vi "Wait and Monitor_UPS.vi"(8 "error in":errorcluster, 10 "Sequence Context":T3, 11 "WaitMoniter Input":T2={"Wait Time(S)"=10.0, "Chamber Temp(Deg C)"=10.0, "Chamber Temp Tolerance(%)"=10.0, "RMS Current(A)"=10.0, "RMS Current Tolerance(%)"=10.0, "Temperature Control"=FALSE, "RMS Control"=FALSE, "RMS Current Min(A)"=10.0, "RMS Current Max(A)"=10.0, "Chamber Temp Min(Deg C)"=10.0, "Chamber Temp Max(Deg C)"=10.0, "HVPPS Current Max(A)"=10.0, "HVPPS Control"=FALSE, "HVPPS Current(A)"=10.0} {"HVPPS Current(A)" format="%#_13g"; "HVPPS Current Max(A)" format="%#_13g"; "Chamber Temp Max(Deg C)" format="%#_13g"; "Chamber Temp Min(Deg C)" format="%#_13g"; "RMS Current Max(A)" format="%#_13g"; "RMS Current Min(A)" format="%#_13g"; "RMS Current Tolerance(%)" format="%#_13g"; "RMS Current(A)" format="%#_13g"; "Chamber Temp Tolerance(%)" format="%#_13g"; "Chamber Temp(Deg C)" format="%#_13g"; "Wait Time(S)" format="%#_13g"}) -> (0 "error out":errorcluster, 2 "Report Text":string, 3 "PowerMoniter out":refnum<class "Wait Monitor.lvclass">)   [LabVIEW 2023, in "HardwareAbstractionLayer_LVOOP.lvlib" / "Wait Monitor.lvclass"]
uses:
  Wait Monitor.lvclass
  <vilib>/addons/TestStand/_TSLegacy.llb/LabVIEW Test - Sequence Context.ctl
  Teststand Steptypes/WaitMoniter/Control/Moniter Step Control.ctl
  SubVI/Control/Data Cluster.ctl
  Teststand Steptypes/PowerMonitor/Control/PowerData.ctl
  SubVI/Control/TimerStates.ctl
  Teststand Steptypes/DAQ/Relay Output/Control/Relay Output.ctl
  <vilib>/addons/TestStand/_TSUtility.llb/TestStand - Get Property Value (Number {Unsigned 16-bit Integer}).vi
  Teststand Steptypes/GlobalVariable/GlobalVariableData.vi
  <vilib>/addons/TestStand/_TSUtility.llb/TestStand - Get Property Value (Number).vi
  <vilib>/addons/TestStand/_TSUtility.llb/TestStand - Set Property Value (Number).vi
  Teststand/Teststand.lvclass
  Teststand Steptypes/LTT_TeststandSteptypes.lvlib
  Database/Database.lvclass
  <userlib>/_OpenG.lib/error/error.llb/openg_error.lvlib
panel:
  out "RMS Refresh?":bool
  out "Elapsed Time":string
  out "HVPPS Current(A)":dbl[](array[numeric]) format="%#.3g"
  out "RTD Temp (Deg C)":dbl
  out "Raw Power":bool
  in  "Buzzer":bool
  out "RMS Current(A)":dbl[](array[numeric]) format="%#.3g"
  out "Target Temp (Deg C)":dbl
  out "Wait Time":string
  out "Current Time":string
  out "Remaining Time":string
  out "Enable Monitor":cluster{"RMS Current":bool, "Chamber":bool}
  out "Running Cycle":u16
  out "Test Mode":u16
  out "PPS Status":T1
  out "RunStates":string
  out "Status Update":string
  out "Elapsed time(S)":dbl format="%.1f"
  out "Chamber Temp(Deg C)":dbl
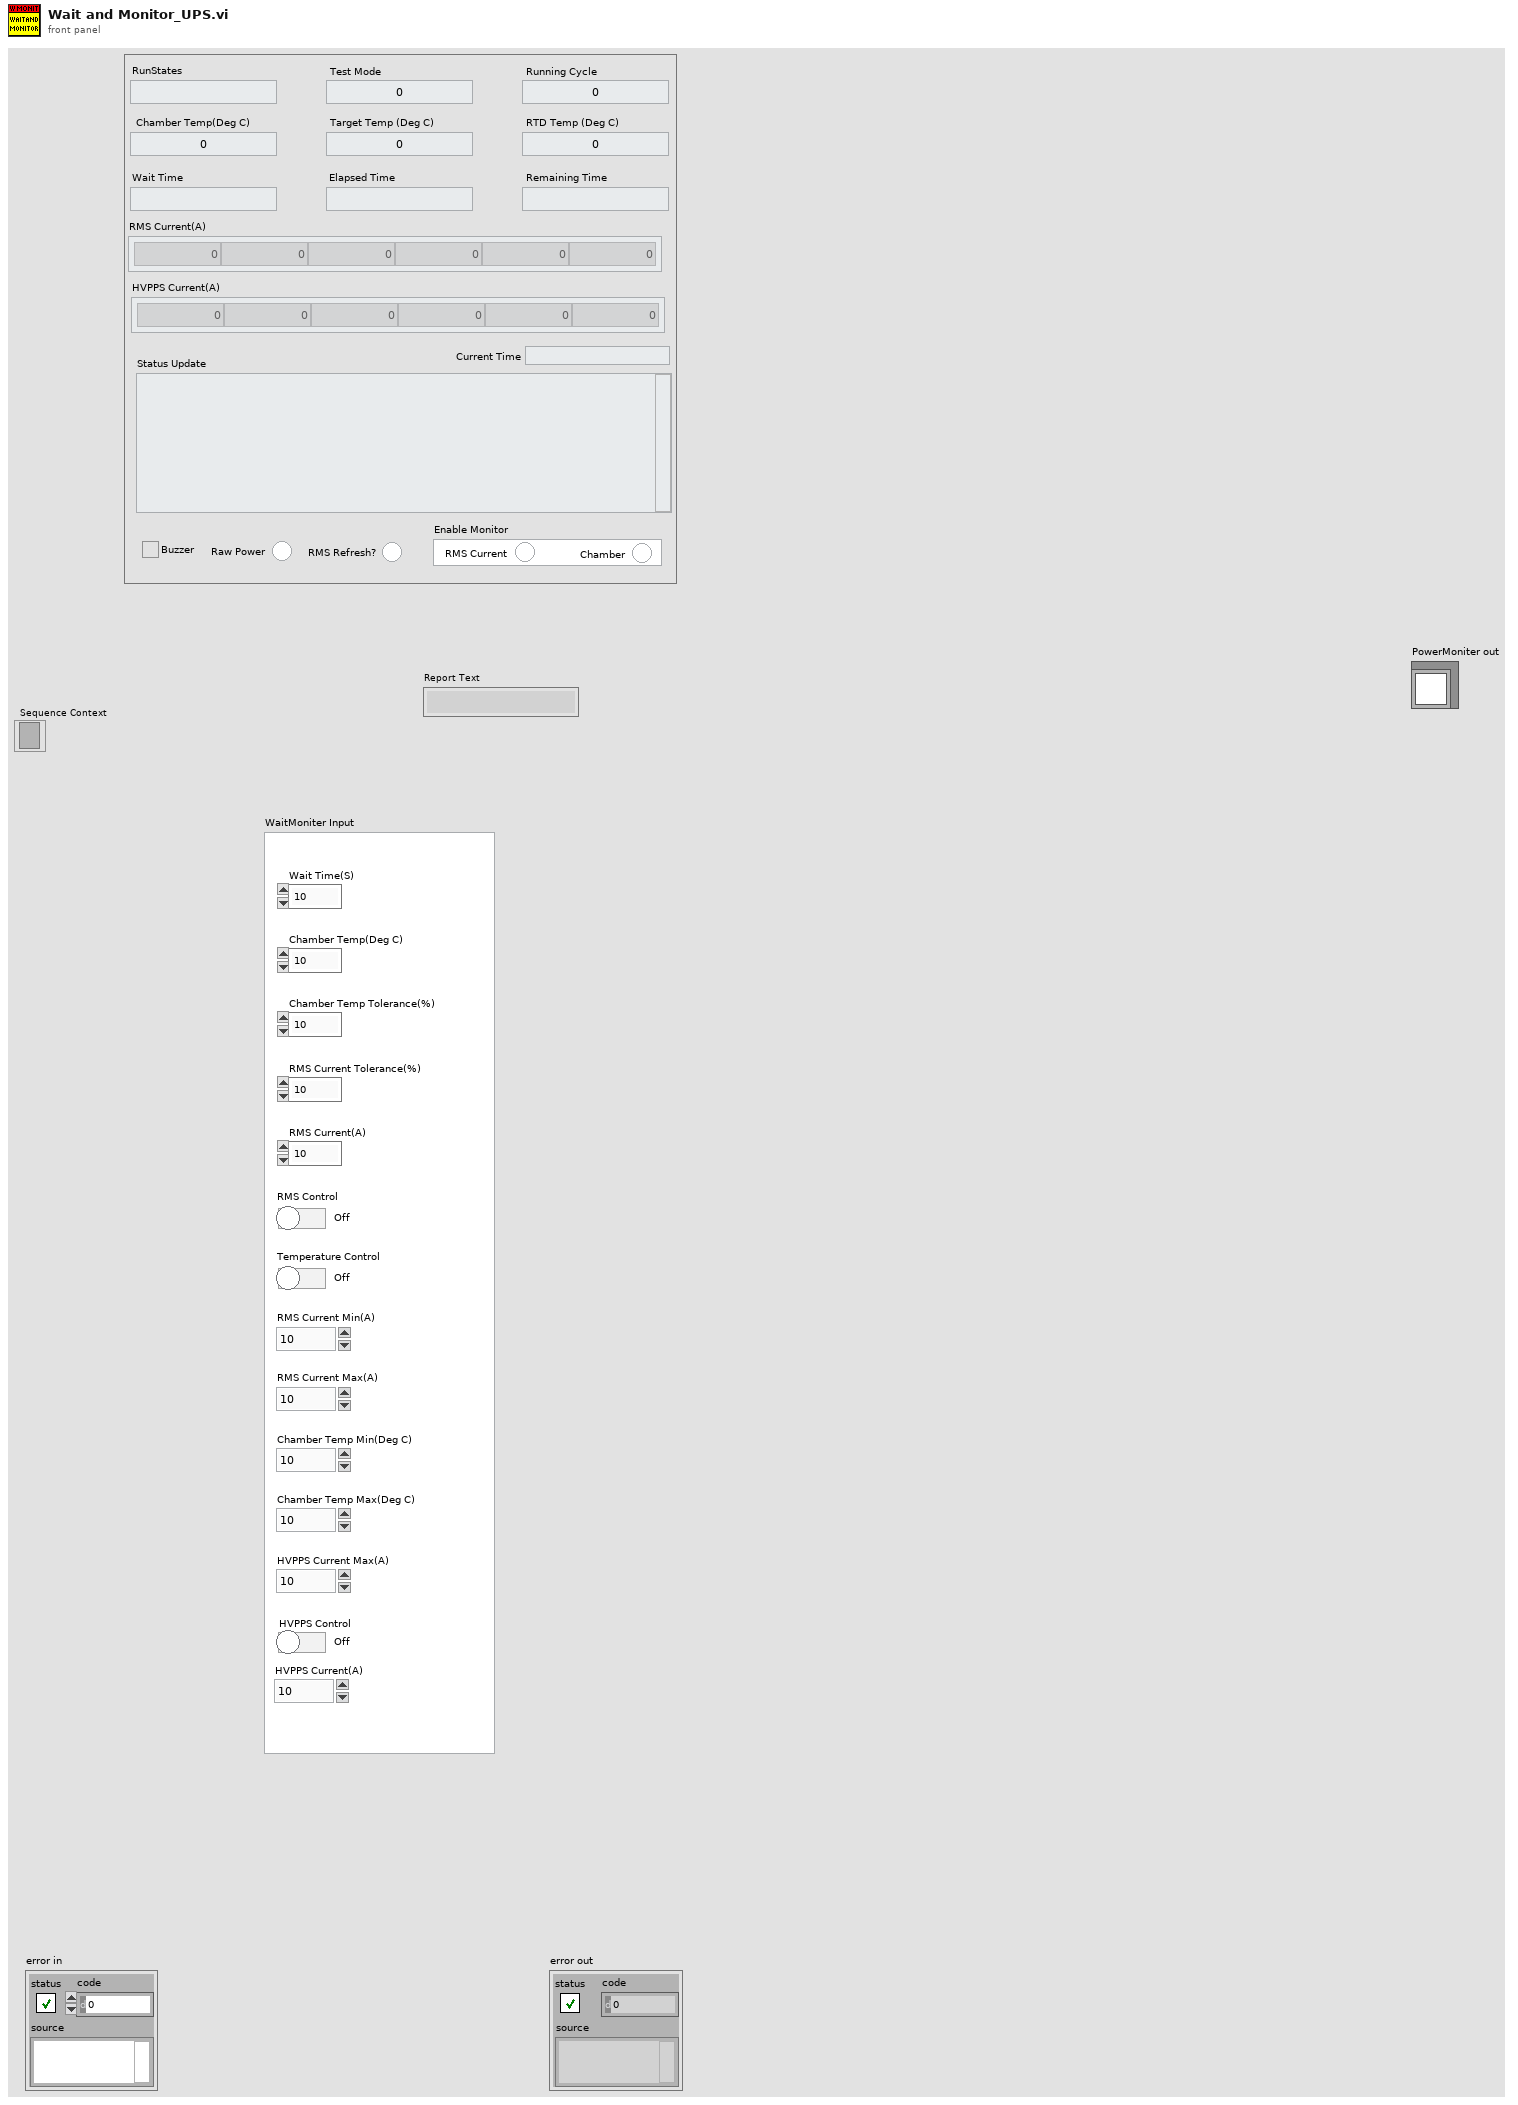
[diagram p1: front panel]
types:
  T1 = cluster{"HV PPS-1":bool, "HV PPS-2":bool, "HV PPS-3":bool, "HV PPS-4":bool, "HV PPS-5":bool, "HV PPS-6":bool, "LV PPS":bool}
  T2 = typedef "HardwareAbstractionLayer_LVOOP.lvlib/Wait Monitor.lvclass/Moniter Step Control.ctl" = cluster{"Wait Time(S)":dbl, "Chamber Temp(Deg C)":dbl, "Chamber Temp Tolerance(%)":dbl, "RMS Current(A)":dbl, "RMS Current Tolerance(%)":dbl, "Temperature Control":bool, "RMS Control":bool, "RMS Current Min(A)":dbl, "RMS Current Max(A)":dbl, "Chamber Temp Min(Deg C)":dbl, "Chamber Temp Max(Deg C)":dbl, "HVPPS Current Max(A)":dbl, "HVPPS Control":bool, "HVPPS Current(A)":dbl}
  T3 = typedef "LabVIEW Test - Sequence Context.ctl" = refnum<k7>
  T4 = typedef "HardwareAbstractionLayer_LVOOP.lvlib/Wait Monitor.lvclass/Data Cluster.ctl" = cluster{"Chamber Address":cluster{"Starting Address":u16, "Data Length":u16}, "Modbus RTU":cluster{"unit ID":u8, "serial type":enum16{"RTU", "ASCII"}, "baud rate":u32, "parity (even)":u16, "flow control (none)":u16, "VISA resource name":refnum<visa-resource-name>}, "Temparature PASS?":bool, "RMS Current PASS?":bool, "Ping PASS?":bool, "WaitMonitor_Class":refnum<class "Wait Monitor.lvclass">, "Status Update":string, "Test Mode":u16, "Sequence Context":T3, "Running?":bool, "RMS_FAIL_Count":u16, "Current Temperature":dbl, "Target Temperature":dbl, "RMS_Current":dbl[], "PowerStatus":T5, "Monitor_Interval(S)":dbl, "Current_Monitor_Interval(S)":dbl, "RMS_Refresh?":bool, "RTD Temperature(Deg C)":dbl, "AbortTime(S)":dbl, "HVPPS_Current":dbl[], "HVPPS Current PASS?":bool}
  T5 = typedef "LTT_TeststandSteptypes.lvlib/PowerData.ctl" = cluster{"Chamber IP Ping":bool, "RAW_Power_Status":bool, "PDU1_Status_Instrument_Rack":bool, "PDU2_Status_PowerSupply_Rack_1":bool, "PDU3_Status_PowerSupply_Rack_2":bool}
  T6 = typedef "TestStand - Status Monitor.ctl" = cluster{"Sequence Context":refnum<k7>, "Execution":refnum<k7>, "Termination Monitor":refnum<k7>}
  T7 = typedef "HardwareAbstractionLayer_LVOOP.lvlib/Wait Monitor.lvclass/TimerStates.ctl" = enum16{"Run", "Pause", "Reset"}
  T8 = cluster{"Set Time":dbl, "Refresh Time":dbl, "RMS_Refresh_Time":dbl}
  T9 = cluster{"Timeout?":bool, "Refresh?":bool, "RMS Refresh?":bool, "Elapsed time":dbl, "Remaining Time":string}
  T10 = typedef "LTT_TeststandSteptypes.lvlib/Relay Output.ctl" = cluster{"Signal Name List":cluster{"Signal Name":string, "Enable Output":bool}[]}
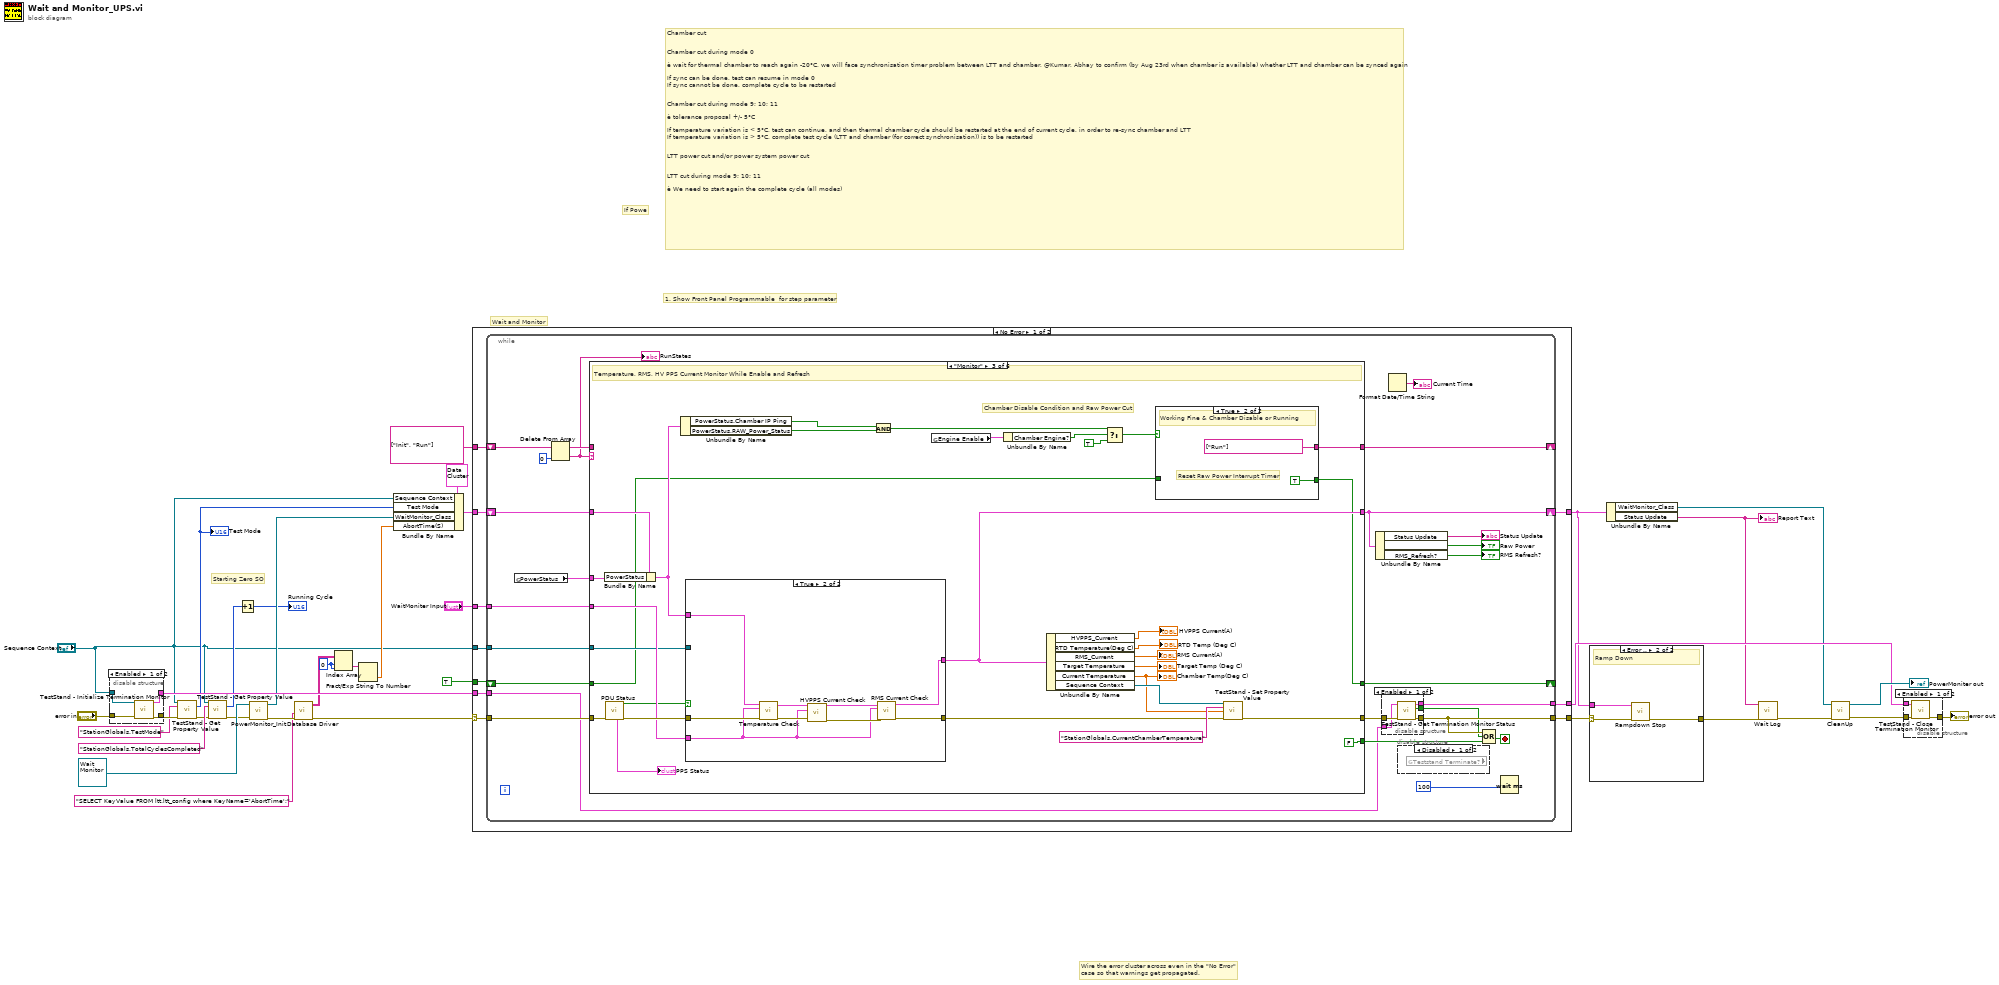
[diagram p0: block diagram]
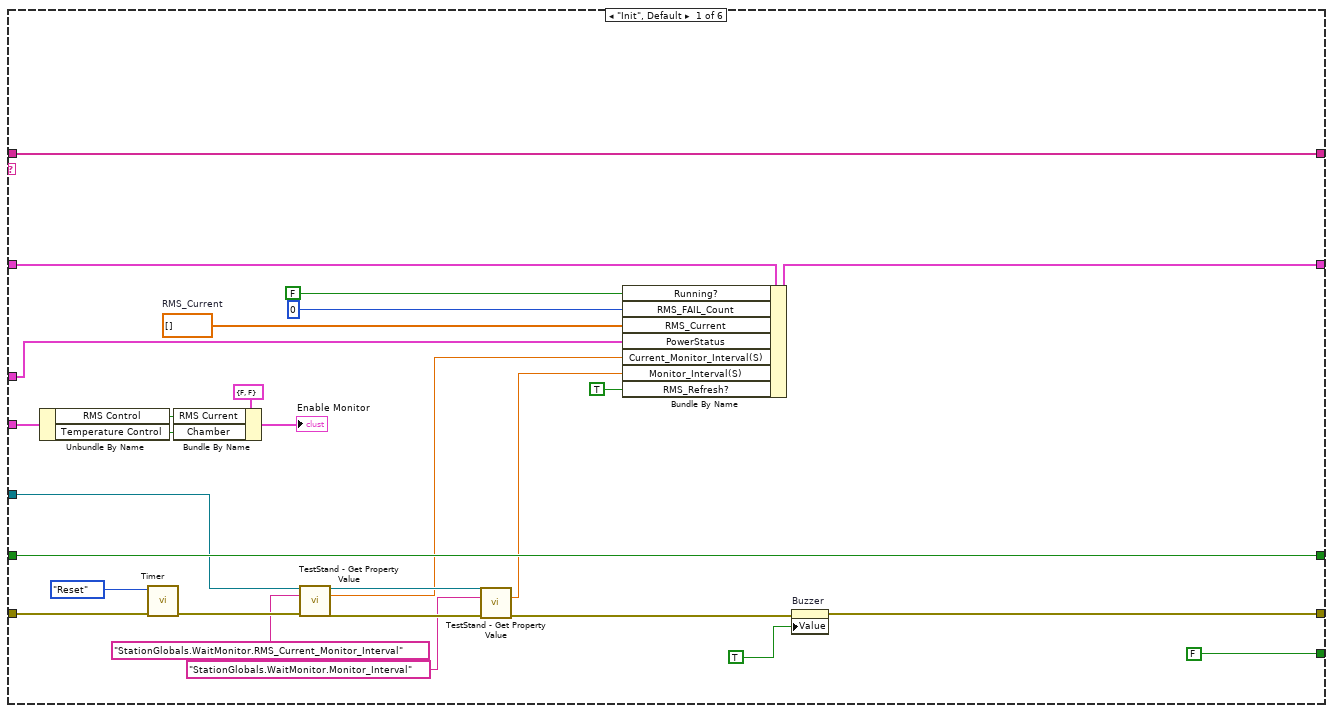
[diagram p7: hidden frame]
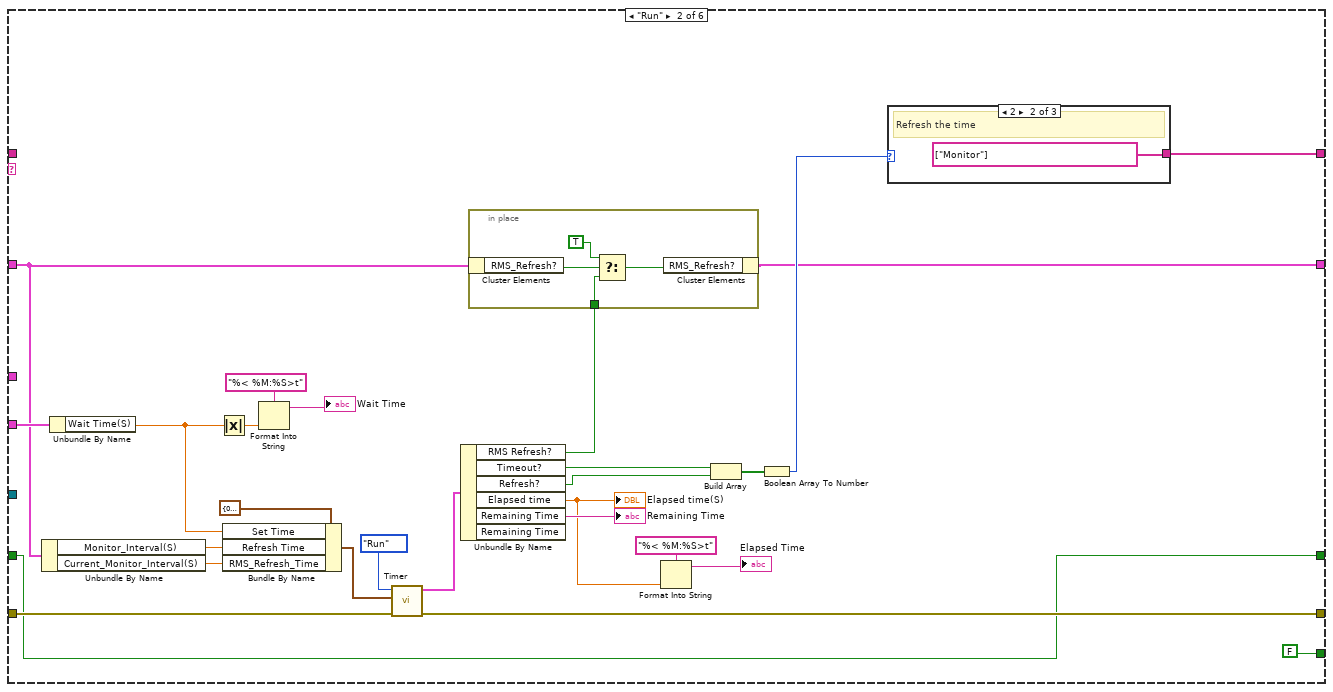
[diagram p8: hidden frame]
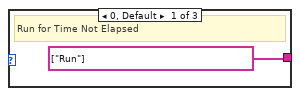
[diagram p9: hidden frame]
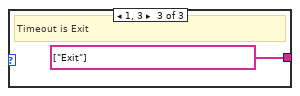
[diagram p10: hidden frame]
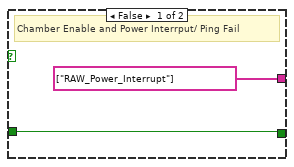
[diagram p11: hidden frame]
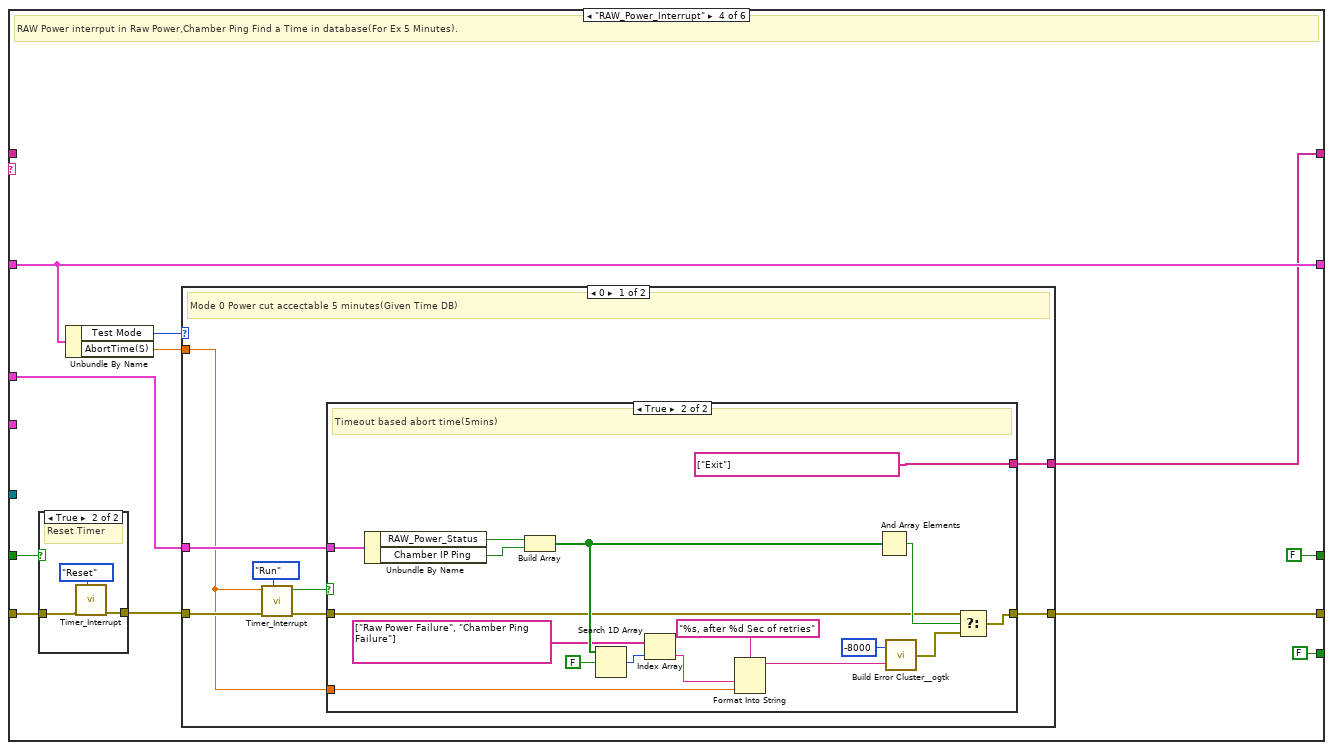
[diagram p13: hidden frame]
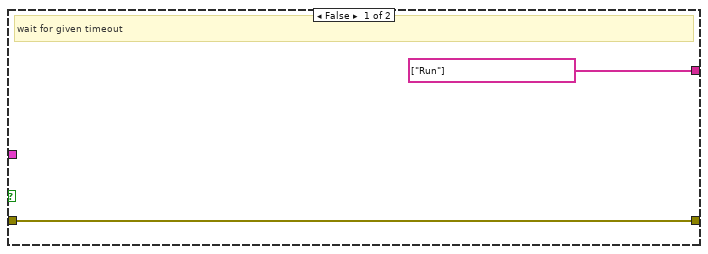
[diagram p15: hidden frame]
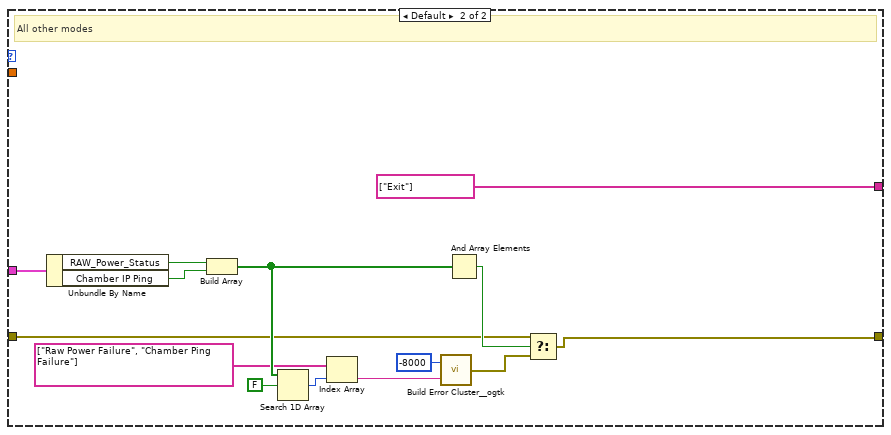
[diagram p16: hidden frame]
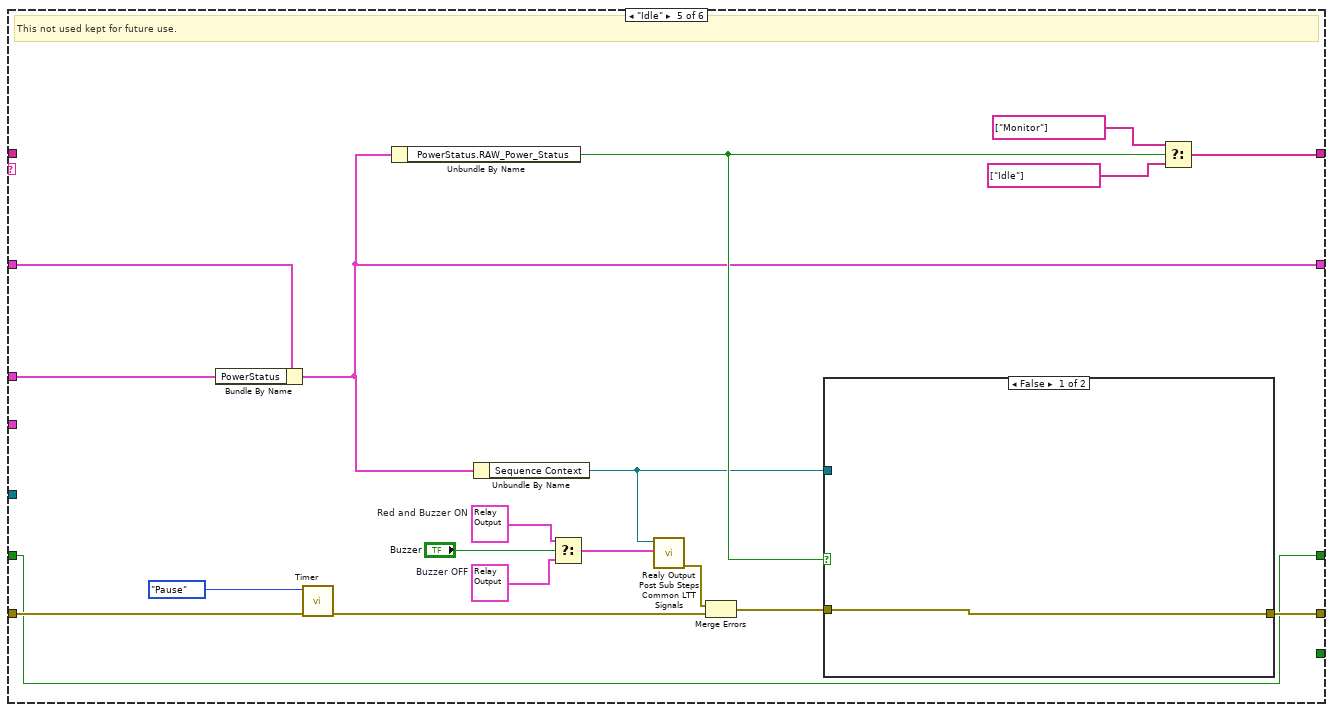
[diagram p17: hidden frame]
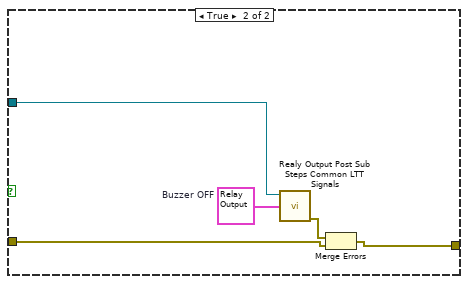
[diagram p18: hidden frame]
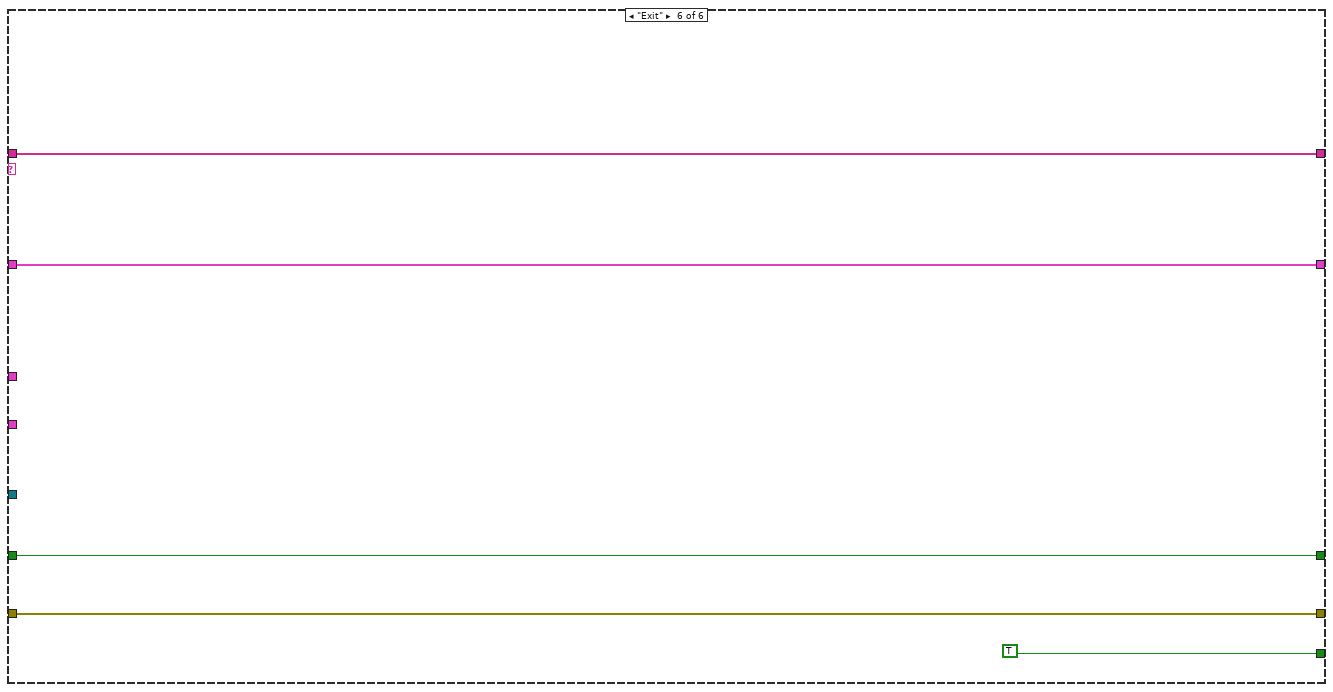
[diagram p19: hidden frame]
diagram:
  w9 = 0 ("index (row)")
  # "Starting Zero SO"
  # "If Powe"
  # "Chamber cut\n \n\nChamber cut during mode 0\n\nè wait for thermal chamber to reach again -20°C, we will face synchronisation timer problem between LTT and chamber, @Kumar, Abhay to confirm (by Aug 23rd when chamber is available) whether LTT and chamber can be synced again\n\nIf sync can be done, test can resume in mode 0\nIf sync cannot be done, complete cycle to be restarted\n \n\nChamber cut during mode 9; 10; 11\n\nè tolerance proposal +/- 5°C\n\nIf temperature variation is < 5°C, test can continue, and then thermal chamber cycle should be restarted at the end of current cycle, in order to re-sync chamber and LTT\nIf temperature variation is > 5°C, complete test cycle (LTT and chamber (for correct synchronisation)) is to be restarted\n \n\nLTT power cut and/or power system power cut\n \n\nLTT cut during mode 9; 10; 11\n\nè We need to start again the complete cycle (all modes)"
  # "1. Show Front Panel Programmable  for step parameter"
  # "Wait and Monitor"
  # "Wire the error cluster across even in the \"No Error\"\ncase so that warnings get propagated."
  n1 = disable-structure shown="Enabled" {
    disable-tunnel: [w39 _] -> w33
    disable-tunnel: "error in" -> [w38 w40]
    disable-tunnel: [w37 w40] -> w26
    disable-tunnel: "Sequence Context" -> [w36 _]
    frame Enabled {
      n2 = call <vilib>:"TestStand - Initialize Termination Monitor.vi"("error in (no error)"=w38, "Sequence Context In"=w36) -> ("error out"=w37:errorcluster, "Status Monitor Out"=w39:T6)  [unwired: 8 in]
    }
    frame Disabled {
    }
  }
  n3 = call-poly <vilib>:"TestStand - Get Property Value.vi"("Sequence Context In"="Sequence Context", "Lookup String"="StationGlobals.TestMode", "error in (no error)"=w26) -> ("Value"=w17:u16, "error out"=w23:errorcluster)  [unwired: 10 in, 1 out]
  "Test Mode" <- w17
  n4 = call-poly <vilib>:"TestStand - Get Property Value.vi"("Sequence Context In"="Sequence Context", "Lookup String"="StationGlobals.TotalCyclesCompleted", "error in (no error)"=w23) -> ("Value"=w21:u16, "error out"=w22:errorcluster)  [unwired: 10 in, 1 out]
  n5 = Increment(x=w21) -> (x+1=→"Running Cycle":u16)
  n6 = call "PowerMonitor_Init.vi"("error in (no error)"=w22, "object in"=refnum<class "Wait Monitor.lvclass"> refnum ("PowerMoniter in")) -> ("error out"=w12:errorcluster, "object out"=w16:refnum<class "Wait Monitor.lvclass">)  [unwired: 8 in]
  n7 = call "Database Driver.vi"("error in"=w12, "SQL query"="SELECT KeyValue FROM ltt.ltt_config where KeyName='AbortTime';") -> ("error out"=w11:errorcluster, "data"=w10:string[][])  [unwired: 6 in, 2 out]
  n8 = Index Array(array=w10, index (row)=w9, index (col)=w9) -> (element=w8:string)
  n9 = Fract/Exp String To Number(string=w8) -> (number=w7:dbl)  [unwired: 3 in, 1 out]
  n10 = Bundle By Name(cluster=T4 {"Chamber Address"={"Starting Address"=0, "Data Length"=0}, "Modbus RTU"={"unit ID"=1, "serial type"=enum."RTU", "baud rate"=9600, "parity (even)"=2, "flow control (none)"=0, "VISA resource name"=""}, "Temparature PASS?"=FALSE, "RMS Current PASS?"=FALSE, "Ping PASS?"=FALSE, "WaitMonitor_Class"=refnum, "Status Update"="", "Test Mode"=0, "Sequence Context"=refnum, "Running?"=FALSE, "RMS_FAIL_Count"=0, "Current Temperature"=0.0, "Target Temperature"=0.0, "RMS_Current"=[], "PowerStatus"={"Chamber IP Ping"=FALSE, "RAW_Power_Status"=FALSE, "PDU1_Status_Instrument_Rack"=FALSE, "PDU2_Status_PowerSupply_Rack_1"=FALSE, "PDU3_Status_PowerSupply_Rack_2"=FALSE}, "Monitor_Interval(S)"=0.0, "Current_Monitor_Interval(S)"=0.0, "RMS_Refresh?"=FALSE, "RTD Temperature(Deg C)"=0.0, "AbortTime(S)"=0.0, "HVPPS_Current"=[], "HVPPS Current PASS?"=FALSE} ("Data Cluster"), "Sequence Context"="Sequence Context", "Test Mode"=w17, "WaitMonitor_Class"=w16, "AbortTime(S)"=w7) -> (w18:T4)
  n11 = case shown="No Error" w11 {
    selector: w11 -> [w50 w277]
    tunnel: [w49 w277] -> w3
    tunnel: w33 -> [w48 w276]
    tunnel: [w47 w276] -> w30
    tunnel: string[] ["Init", "Run"] -> [w46 _]
    tunnel: w18 -> [w45 w275]
    tunnel: "WaitMoniter Input" -> [w44 _]
    tunnel: [w43 w275] -> w1
    tunnel: TRUE -> [w42 _]
    tunnel: "Sequence Context" -> [w41 _]
    frame No Error {
      n12 = while {
        tunnel: w50 -> [w75]
        tunnel: [w65] -> w49
        tunnel: w48 -> [w64]
        tunnel: [w72] -> w47
        shift-right: [w69] -> _
        shift-left: w46 -> [w71]
        tunnel: w44 -> [w66]
        shift-right: [w60] -> w43
        shift-left: w45 -> [w67]
        shift-right: [w55] -> _
        shift-left: w42 -> [w56]
        tunnel: w41 -> [w54]
        stop <- w68 stop-if-true
        n13 = global read "GlobalVariableData.vi" "PowerStatus"() -> (w57:T5)
        n14 = Delete From Array(array=w71, index=0) -> (deleted portion=w63:string, array with subset deleted=w70:string[])  [unwired: 1 in]
        "RunStates" <- w63
        n15 = case shown="\"Monitor\"" w63 {
          tunnel: w75 -> [w94 w133 w170 w191 w259 w271]
          tunnel: [w97 w128 w153 w197 w249 w271] -> w73
          tunnel: [FALSE FALSE FALSE FALSE _ TRUE] -> w74
          tunnel: w70 -> [w108 _ _ _ _ w273]
          tunnel: [w108 w132 w166 w194 w260 w273] -> w69
          tunnel: w67 -> [w107 w116 w158 w196 w252 w272]
          tunnel: w66 -> [w106 w134 w171 _ _ _]
          tunnel: [w101 w114 w160 w196 w246 w272] -> w60
          tunnel: w57 -> [w95 _ w159 w198 w251 _]
          tunnel: w56 -> [w91 w113 w145 w189 w245 w270]
          tunnel: [w91 w113 w144 FALSE w245 w270] -> w55
          tunnel: w54 -> [w90 _ w151 _ _ _]
          frame "Init", Default {
            w98 = dbl[] []  # RMS_Current
            n16 = Unbundle By Name(w106) -> ("RMS Control"=w103:bool, "Temperature Control"=w102:bool)
            n17 = call "Timer.vi"("error in"=w94, "Options"=TimerStates."Reset") -> ("error out"=w89:errorcluster)  [unwired: 8 in, 1 out]
            n18 = Bundle By Name(cluster=cluster{"RMS Current":bool, "Chamber":bool} {"RMS Current"=FALSE, "Chamber"=FALSE} ("Enable Monitor"), "RMS Current"=w103, "Chamber"=w102) -> (→"Enable Monitor":cluster{"RMS Current":bool, "Chamber":bool})
            n19 = call-poly <vilib>:"TestStand - Get Property Value.vi"("Sequence Context In"=w90, "Lookup String"="StationGlobals.WaitMonitor.RMS_Current_Monitor_Interval", "error in (no error)"=w89) -> ("Sequence Context Out"=w87:refnum<k7>, "Value"=w83:dbl, "error out"=w86:errorcluster)  [unwired: 10 in]
            n20 = call-poly <vilib>:"TestStand - Get Property Value.vi"("Sequence Context In"=w87, "Lookup String"="StationGlobals.WaitMonitor.Monitor_Interval", "error in (no error)"=w86) -> ("Value"=w82:dbl, "error out"=w84:errorcluster)  [unwired: 10 in, 1 out]
            n21 = Bundle By Name(cluster=w107, "Running?"=FALSE, "RMS_FAIL_Count"=u16 0, "RMS_Current"=w98, "PowerStatus"=w95, "Current_Monitor_Interval(S)"=w83, "Monitor_Interval(S)"=w82, "RMS_Refresh?"=TRUE) -> (w101:T4)
            n22 = property on="Buzzer" class="Bool (strict)"(error in=w84, "Value"=TRUE ("Buzzer")) -> (error out=w97:errorcluster)  [unwired: 1 in, 1 out]
          }
          frame "Run" {
            n23 = Unbundle By Name(w116) -> ("Monitor_Interval(S)"=w122:dbl, "Current_Monitor_Interval(S)"=w121:dbl)
            n24 = Unbundle By Name(w134) -> ("Wait Time(S)"=w123:dbl)
            n25 = Absolute Value(x=w123) -> (abs(x)=w131:dbl)
            n26 = Bundle By Name(cluster=T8 {"Set Time"=0.0, "Refresh Time"=0.0, "RMS_Refresh_Time"=0.0} ("Input Data"), "Set Time"=w123, "Refresh Time"=w122, "RMS_Refresh_Time"=w121) -> (w120:T8)
            n27 = Format Into String(format string="%< %M:%S>t", w131) -> (resulting string=→"Wait Time":string)  [unwired: 2 in, 1 out]
            n28 = call "Timer.vi"("error in"=w133, "Input Data"=w120, "Options"=TimerStates."Run") -> ("error out"=w128:errorcluster, "Output Data"=w127:T9)  [unwired: 7 in]
            n29 = Unbundle By Name(w127) -> ("RMS Refresh?"=w115:bool, "Timeout?"=w119:bool, "Refresh?"=w118:bool, "Elapsed time"=w111:dbl, "Remaining Time"=→"Remaining Time":string)  [unwired: 1 out]
            "Elapsed time(S)" <- w111
            n30 = in-place {
              in-place-border: w115 -> [w139]
              n31 = in-place-cluster #1(w116) -> ("RMS_Refresh?"=w140:bool)
              n32 = Select(t=TRUE, s=w140, f=w139) -> (s? t:f=w137:bool)
              n33 = in-place-cluster #1("RMS_Refresh?"=w137) -> (w114:T4)
            }
            n34 = Format Into String(format string="%< %M:%S>t", w111) -> (resulting string=→"Elapsed Time":string)  [unwired: 2 in, 1 out]
            n35 = Build Array(w119, w118) -> (w126:bool[])
            n36 = Boolean Array To Number(Boolean array=w126) -> (number=w125:u32)
            n37 = case shown="2" w125 {
              tunnel: [string[] ["Run"] string[] ["Monitor"] string[] ["Exit"]] -> w132
              frame 0, Default {
                # "Run for Time Not Elapsed"
              }
              frame 2 {
                # "Refresh the time"
              }
              frame 1, 3 {
                # "Timeout is Exit"
              }
            }
          }
          frame "Monitor" {
            # "Chamber Disable Condition and Raw Power Cut"
            # "Temperature, RMS, HV PPS Current Monitor While Enable and Refresh"
            n38 = Bundle By Name(cluster=w158, "PowerStatus"=w159) -> (w157:T4)
            n39 = call "PDU Status.vi"("error in"=w170) -> ("error out"=w172:errorcluster, "OK"=w165:bool, "PPS Status"=→"PPS Status":T1)  [unwired: 7 in, 1 out]
            n40 = Unbundle By Name(w157) -> ("PowerStatus.Chamber IP Ping"=w155:bool, "PowerStatus.RAW_Power_Status"=w154:bool)
            n41 = case shown="True" w165 {
              tunnel: w172 -> [w179 w188]
              tunnel: w157 -> [w178 w187]
              tunnel: w171 -> [_ w180]
              tunnel: [w179 w186] -> w167
              tunnel: [w178 w185] -> w160
              tunnel: w151 -> [_ _]
              frame False {
                # "Temperature Updates"
              }
              frame True {
                n42 = call "Temperature Check.vi"("error in (no error)"=w188, "WaitMoniter Input"=w180, "Data Cluster"=w187) -> ("error out"=w184:errorcluster, "Data Cluster out"=w183:T4)  [unwired: 7 in]
                n43 = call "HVPPS Current Check.vi"("error in"=w184, "WaitMoniter Input"=w180, "Data Cluster"=w183) -> ("error out"=w181:errorcluster, "Data Cluster out"=w182:T4)  [unwired: 7 in]
                n44 = call "RMS Current Check.vi"("error in"=w181, "WaitMoniter Input"=w180, "Data Cluster"=w182) -> ("error out"=w186:errorcluster, "Data Cluster out"=w185:T4)  [unwired: 7 in]
              }
            }
            n45 = And(x=w155, y=w154) -> (x .and. y?=w147:bool)
            n46 = global read "GlobalVariableData.vi" "Engine Enable"() -> (w149:cluster{"Chamber Engine?":bool})
            n47 = Unbundle By Name(w149) -> ("Chamber Engine?"=w148:bool)
            n48 = Unbundle By Name(w160) -> ("HVPPS_Current"=→"HVPPS Current(A)":dbl[], "RTD Temperature(Deg C)"=→"RTD Temp (Deg C)":dbl, "RMS_Current"=→"RMS Current(A)":dbl[], "Target Temperature"=→"Target Temp (Deg C)":dbl, "Current Temperature"=w163:dbl, "Sequence Context"=w164:T3)
            "Chamber Temp(Deg C)" <- w163
            n49 = Select(t=w147, s=w148, f=TRUE) -> (s? t:f=w150:bool)
            n50 = case shown="True" w150 {
              tunnel: [string[] ["RAW_Power_Interrupt"] string[] ["Run"]] -> w166
              tunnel: w145 -> [w174 _]
              tunnel: [w174 TRUE] -> w144
              frame False {
                # "Chamber Enable and Power Interrput/ Ping Fail"
              }
              frame True {
                # "Reset Raw Power Interrupt Timer"
                # "Working Fine & Chamber Disable or Running"
              }
            }
            n51 = call-poly <vilib>:"TestStand - Set Property Value.vi"("Sequence Context In"=w164, "Lookup String"="StationGlobals.CurrentChamberTemperature", "New Value"=w163, "error in (no error)"=w167) -> ("error out"=w153:errorcluster)  [unwired: 10 in, 1 out]
          }
          frame "RAW_Power_Interrupt" {
            # "RAW Power interrput in Raw Power,Chamber Ping Find a Time in database(For Ex 5 Minutes)."
            n52 = case shown="True" w189 {
              tunnel: w191 -> [w200 w202]
              tunnel: [w200 w201] -> w190
              frame False {
              }
              frame True {
                # "Reset Timer"
                n53 = call "Timer_Interrupt.vi"("Options"=TimerStates."Reset", "error in"=w202) -> ("error out"=w201:errorcluster)  [unwired: 8 in, 1 out]
              }
            }
            n54 = Unbundle By Name(w196) -> ("Test Mode"=w195:u16, "AbortTime(S)"=w193:dbl)
            n55 = case shown="0" w195 {
              tunnel: w198 -> [w209 w242]
              tunnel: [w211 w244] -> w197
              tunnel: w190 -> [w208 w232]
              tunnel: [w210 string[] ["Exit"]] -> w194
              tunnel: w193 -> [w204 _]
              frame 0 {
                # "Mode 0 Power cut accectable 5 minutes(Given Time DB)"
                n56 = call "Timer_Interrupt.vi"("Options"=TimerStates."Run", "error in"=w208, "Set Time"=w204) -> ("error out"=w207:errorcluster, "Elapsed?"=w206:bool)  [unwired: 7 in]
                n57 = case shown="True" w206 {
                  tunnel: w207 -> [w212 w222]
                  tunnel: [w212 w221] -> w211
                  tunnel: [string[] ["Run"] string[] ["Exit"]] -> w210
                  tunnel: w209 -> [_ w223]
                  tunnel: w204 -> [_ w215]
                  frame False {
                    # "wait for given timeout"
                  }
                  frame True {
                    # "Timeout based abort time(5mins)"
                    n58 = Unbundle By Name(w223) -> ("RAW_Power_Status"=w228:bool, "Chamber IP Ping"=w227:bool)
                    n59 = Build Array(w228, w227) -> (w225:bool[])
                    n60 = Search 1D Array(1D array=w225, element=FALSE) -> (index of element=w220:i32)  [unwired: 1 in]
                    n61 = Index Array(array=string[] ["Raw Power Failure", "Chamber Ping Failure"], index=w220) -> (element=w216:string)
                    n62 = Format Into String(format string="%s, after %d Sec of retries", w216, w215) -> (resulting string=w214:string)  [unwired: 2 in, 1 out]
                    n63 = And Array Elements(Boolean array=w225) -> (logical AND=w226:bool)
                    n64 = call <userlib>:"Build Error Cluster__ogtk.vi"("String to Prepend to source (\"\")"=w214, "code"=-8000) -> ("error out"=w229:errorcluster)
                    n65 = Select(t=w222, s=w226, f=w229) -> (s? t:f=w221:errorcluster)
                  }
                }
              }
              frame Default {
                # "All other modes"
                n66 = Unbundle By Name(w242) -> ("RAW_Power_Status"=w240:bool, "Chamber IP Ping"=w239:bool)
                n67 = Build Array(w240, w239) -> (w237:bool[])
                n68 = Search 1D Array(1D array=w237, element=FALSE) -> (index of element=w235:i32)  [unwired: 1 in]
                n69 = Index Array(array=string[] ["Raw Power Failure", "Chamber Ping Failure"], index=w235) -> (element=w231:string)
                n70 = call <userlib>:"Build Error Cluster__ogtk.vi"("String to Prepend to source (\"\")"=w231, "code"=-8000) -> ("error out"=w241:errorcluster)
                n71 = And Array Elements(Boolean array=w237) -> (logical AND=w238:bool)
                n72 = Select(t=w232, s=w238, f=w241) -> (s? t:f=w244:errorcluster)
              }
            }
          }
          frame "Idle" {
            w254 = T10 {"Signal Name List"=[{"Signal Name"="TL Green", "Enable Output"=FALSE}, {"Signal Name"="TL Red", "Enable Output"=TRUE}, {"Signal Name"="TL Yellow", "Enable Output"=FALSE}, {"Signal Name"="TL Buzzer", "Enable Output"=FALSE}]}  # Buzzer OFF
            w256 = T10 {"Signal Name List"=[{"Signal Name"="TL Green", "Enable Output"=FALSE}, {"Signal Name"="TL Red", "Enable Output"=TRUE}, {"Signal Name"="TL Yellow", "Enable Output"=FALSE}, {"Signal Name"="TL Buzzer", "Enable Output"=TRUE}]}  # Red and Buzzer ON
            # "This not used kept for future use."
            n73 = Bundle By Name(cluster=w252, "PowerStatus"=w251) -> (w246:T4)
            n74 = call "Timer.vi"("error in"=w259, "Options"=TimerStates."Pause") -> ("error out"=w258:errorcluster)  [unwired: 8 in, 1 out]
            n75 = Unbundle By Name(w246) -> ("PowerStatus.RAW_Power_Status"=w248:bool)
            n76 = Unbundle By Name(w246) -> ("Sequence Context"=w247:T3)
            n77 = Select(t=w256, s="Buzzer", f=w254) -> (s? t:f=w255:T10)
            n78 = call "Realy Output Post Sub Steps Common LTT Signals.vi"("RelayOutputWrite"=w255, "Sequence Context In"=w247) -> ("error out"=w263:errorcluster)  [unwired: 7 in, 2 out]
            n79 = Merge Errors(w263, w258) -> (w250:errorcluster)
            n80 = case shown="False" w248 {
              tunnel: w250 -> [w264 w269]
              tunnel: [w264 w267] -> w249
              tunnel: w247 -> [_ w266]
              frame False {
              }
              frame True {
                w265 = T10 {"Signal Name List"=[{"Signal Name"="TL Green", "Enable Output"=TRUE}, {"Signal Name"="TL Red", "Enable Output"=FALSE}, {"Signal Name"="TL Yellow", "Enable Output"=FALSE}, {"Signal Name"="TL Buzzer", "Enable Output"=FALSE}]}  # Buzzer OFF
                n81 = call "Realy Output Post Sub Steps Common LTT Signals.vi"("RelayOutputWrite"=w265, "Sequence Context In"=w266) -> ("error out"=w268:errorcluster)  [unwired: 7 in, 2 out]
                n82 = Merge Errors(w268, w269) -> (w267:errorcluster)
              }
            }
            n83 = Select(t=string[] ["Monitor"] ("f"), s=w248, f=string[] ["Idle"]) -> (s? t:f=w260:string[])
          }
          frame "Exit" {
          }
        }
        n84 = Unbundle By Name(w60) -> ("Status Update"=→"Status Update":string, "PowerStatus.RAW_Power_Status"=→"Raw Power":bool, "RMS_Refresh?"=→"RMS Refresh?":bool)
        n85 = disable-structure shown="Enabled" {
          disable-tunnel: w73 -> [w80 w81]
          disable-tunnel: [w79 _] -> w72
          disable-tunnel: [w78 w81] -> w65
          disable-tunnel: w64 -> [w77 _]
          disable-tunnel: [w76 _] -> w53
          frame Enabled {
            n86 = call <vilib>:"TestStand - Get Termination Monitor Status.vi"("error in (no error)"=w80, "Status Monitor In"=w77) -> ("error out"=w78:errorcluster, "Terminating or Aborting"=w76:bool, "Status Monitor Out"=w79:T6)  [unwired: 7 in]
          }
          frame Disabled {
          }
        }
        n87 = Format Date/Time String() -> (date/time string=→"Current Time":string)  [unwired: 3 in]
        n88 = disable-structure shown="Disabled" {
          frame Disabled {
            n89 = global read "GlobalVariableData.vi" "Teststand Terminate?"() -> ()  [unwired: 1 out]
          }
          frame Enabled {
          }
        }
        n90 = Compound Arithmetic op=OR(w65, w53, w74) -> (w68:bool)
        n91 = Wait (ms)(milliseconds to wait=u32 100 ("millisecond multiple")) -> ()  [unwired: 1 out]
      }
    }
    frame Error {
    }
  }
  n92 = case shown="Error .." w3 {
    selector: w3 -> [w278 w281]
    tunnel: [w278 w280] -> w2
    tunnel: w1 -> [_ w279]
    frame No Error {
    }
    frame Error {
      # "Ramp Down"
      n93 = call "Rampdown Stop.vi"("error in"=w281, "Data Cluster"=w279) -> ("error out"=w280:errorcluster)  [unwired: 8 in, 1 out]
    }
  }
  n94 = Unbundle By Name(w1) -> ("WaitMonitor_Class"=w14:refnum<class "Wait Monitor.lvclass">, "Status Update"=w15:string)
  "Report Text" <- w15
  n95 = call "Wait Log.vi"("error in"=w2, "Log Data"=w15) -> ("error out"=w20:errorcluster)  [unwired: 9 in]
  n96 = call-dynamic "CleanUp.vi"("error in (no error)"=w20, "object in"=w14) -> ("error out"=w32:errorcluster, "object out"=→"PowerMoniter out":refnum<class "Wait Monitor.lvclass">)  [unwired: 8 in]
  n97 = disable-structure shown="Enabled" {
    disable-tunnel: w32 -> [w284 w285]
    disable-tunnel: [w283 w285] -> w31
    disable-tunnel: w30 -> [w282 _]
    frame Enabled {
      n98 = call <vilib>:"TestStand - Close Termination Monitor.vi"("error in (no error)"=w284, "Status Monitor In"=w282) -> ("error out"=w283:errorcluster)  [unwired: 9 in]
    }
    frame Disabled {
    }
  }
  "error out" <- w31
